vi "writeToFIFO.vi"() -> ()   [LabVIEW 2012]
uses:
  <vilib>/Utility/file.llb/Read From Spreadsheet File (I64).vi
  <vilib>/Analysis/Matrix/Numeric/Conversions/Matrix To Array - RM.vi
  <vilib>/FPGAPlugInAG/cRIO-9082/niLvFpga_Open_cRIO-9082.vi
  <vilib>/rvi/interface/common/dynamic/niFpgaDynamicAddResources.vi
  <vilib>/FPGAPlugInAG/Dynamic/niLvFpga_Reset_Dynamic.vi
  <vilib>/Utility/error.llb/Error Cluster From Error Code.vi
  <vilib>/rvi/errors/niLvFpgaAdjustHostInterfaceError.vi
  <vilib>/FPGAPlugInAG/Dynamic/niLvFpga_Run_Dynamic.vi
  <vilib>/FPGAPlugInAG/Dynamic/niLvFpga_Abort_Dynamic.vi
  <vilib>/rvi/interface/nirviOpenFPGA/nirviOpenFPGA.xnode
  FPGA Bitfiles/simpletest_FPGATarget_test3_auvyVXmVhlg.lvbitx
  <vilib>/rvi/interface/nirviMethod/nirviMethod.xnode
  <vilib>/rvi/interface/nirviReadWriteControl/nirviReadWriteControl.xnode
  <vilib>/Analysis/Matrix/NI_Matrix.lvlib
  <vilib>/rvi/errors/niLvFpgaMergeErrorWithErrorCode.vi
  <vilib>/FPGAPlugInAG/Dynamic/niLvFpga_WriteFifo_Dynamic.vi
  NiFpgaLv.dll
  <vilib>/rvi/interface/Simulation/niFpgaSimulationCallBeginRW.vi
  <vilib>/FPGAPlugInAG/Dynamic/niLvFpga_ConfigureFifo_Dynamic.vi
panel:
  out "Actual Depth":u32
  out "RemaingSpace":u32
  out "ToRead":u32
  out "x_pos":u16
  out "y_pos":u16
  out "length":u16
  out "direction":u16
  out "all rows":i64[][](array[numeric])
  out "row":i32
  out "col":i32
  out "size":i32
  out "input array":u16[](array[numeric])
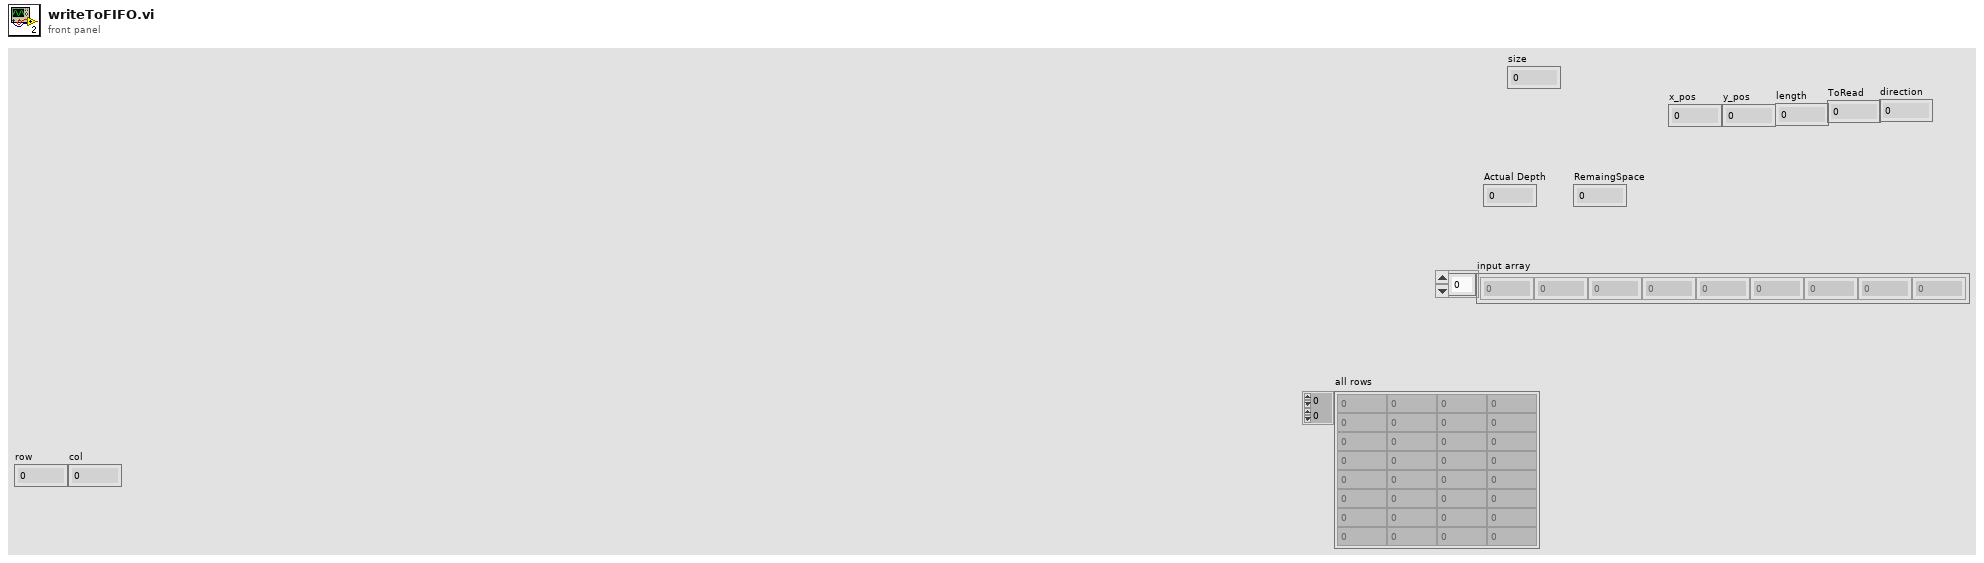
[diagram p1: front panel]
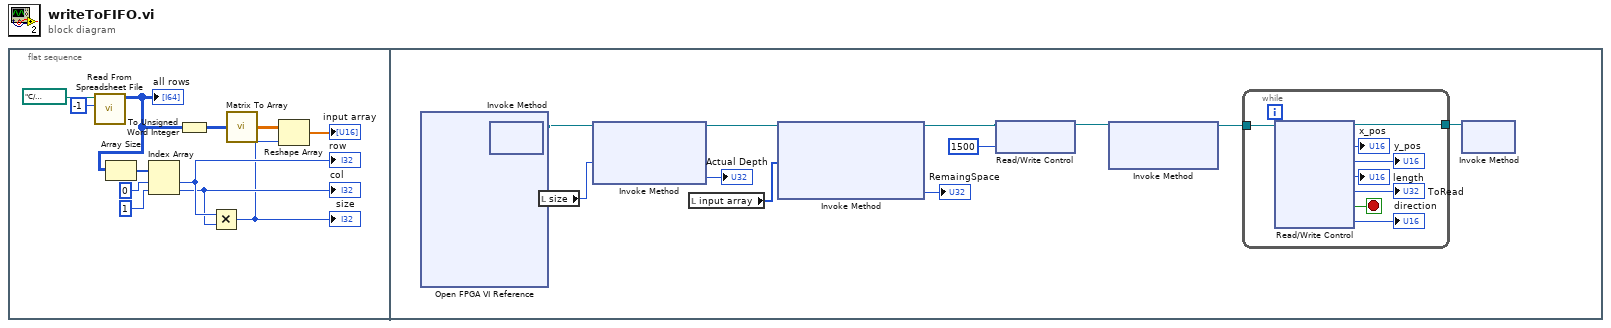
[diagram p0: block diagram]
diagram:
  n1 = flat-sequence {
    frame #0 {
      n2 = call-poly <vilib>:"Read From Spreadsheet File.vi"("number of rows (all:-1)"=-1, "file path (dialog if empty)"=path "C:/Documents and Settings/Owner/Desktop/yufan/path trajectory/upathlocations.txt") -> ("all rows"=w5:i64[][])  [unwired: 5 in, 4 out]
      "all rows" <- w5
      n3 = Array Size(array=w5) -> (size(s)=w10:i32[])
      n4 = Index Array(array=w10, index #1=0 ("index"), index #2=1 ("index")) -> (element #1=w7:i32, element #2=w6:i32)
      "row" <- w7
      "col" <- w6
      n5 = To Unsigned Word Integer(number=w5) -> (unsigned 16bit integer=w4:u16[][])
      n6 = Multiply(x=w7, y=w6) -> (x*y=w2:i32)
      "size" <- w2
      n7 = call-poly <vilib>:"Matrix To Array.vi"("Real Matrix"=w4) -> ("Real 2D Array"=w3:dbl[][])
      n8 = Reshape Array(w3, w2) -> (→"input array":dbl[])
    }
    frame #1 {
      n9 = xnode "Open FPGA VI Reference"() -> ("FPGA VI Reference Out"=w24:refnum<k20>)  [unwired: 2 in, 1 out]
      n10 = xnode "Invoke Method"("FPGA VI Reference In"=w24) -> ("FPGA VI Reference Out"=w23:refnum<k20>)  [unwired: 1 in, 1 out]
      n11 = local read "size"() -> (w19:i32)
      n12 = xnode "Invoke Method"("FPGA VI Reference In"=w23, "Requested Depth"=w19) -> ("FPGA VI Reference Out"=w18:refnum<k20>, "Actual Depth"=→"Actual Depth":u32)  [unwired: 1 in, 1 out]
      n13 = local read "input array"() -> (w21:u16[])
      n14 = xnode "Invoke Method"("FPGA VI Reference In"=w18, "Data"=w21) -> ("FPGA VI Reference Out"=w15:refnum<k20>, "Empty Elements Remaining"=→"RemaingSpace":u32)  [unwired: 2 in, 1 out]
      n15 = xnode "Read/Write Control"("FPGA VI Reference In"=w15, "Clock (mSec)"=u32 1500) -> ("FPGA VI Reference Out"=w14:refnum<k20>)  [unwired: 1 in, 1 out]
      n16 = xnode "Invoke Method"("FPGA VI Reference In"=w14) -> ("FPGA VI Reference Out"=w16:refnum<k20>)  [unwired: 2 in, 1 out]
      n17 = while {
        tunnel: [w27] -> w17
        tunnel: w16 -> [w26]
        stop <- w28 stop-if-true
        n18 = xnode "Read/Write Control"("FPGA VI Reference In"=w26) -> ("FPGA VI Reference Out"=w27:refnum<k20>, "x_pos"=→"x_pos":u16, "y_pos"=→"y_pos":u16, "length"=→"length":u16, "ToRead"=→"ToRead":u32, "signalToStop"=w28:bool, "direction"=→"direction":u16)  [unwired: 1 in, 1 out]
      }
      n19 = xnode "Invoke Method"("FPGA VI Reference In"=w17) -> ()  [unwired: 1 in, 2 out]
    }
  }
